vi "stabilizePress_06.vi"() -> ()   [LabVIEW 2011]
uses:
  <vilib>/Analysis/NI_AALPro.lvlib
panel:
  out "dt_array":dbl[](array[numeric])
  out "P_i+1 (torr)":dbl=20.01 caption="P_i+1(torr)" format="%.2f"
  out "Polynomial Coefficients":dbl[](array[numeric])
  in  "n":dbl
  in  "points":i32
  out "P array":dbl[](array[numeric])
  out "t array":dbl[](array[numeric])
  in  "i":u16
  out "tElaps":dbl=32.29700000002049
  in  "dT_fit(s)":dbl=1.0
  in  "tTotal(s)":dbl=30.0
  out "XY Graph":cluster{"Value":dbl[], "Value":dbl[]}(graph)={"Value"=[1.5420000000158325, 3.0790000000270084, 4.619000000006054, 6.157000000006519, 7.695000000006985, 9.23300000000745, 10.772999999986496, 12.309999999997672, 13.847000000008848, 15.386999999987893, 16.92399999999907, 18.462999999988824, 19.99900000001071, 21.53499999997439, 23.07400000002235, 24.61099999997532, 26.147999999986496, 27.68499999999767, 29.222999999998137, 30.760999999998603, 32.29700000002049], "Value"=[16.36, 19.38, 18.91, 17.669999999999998, 16.93, 17.98, 18.610000000000003, 18.83, 19.259999999999998, 19.459999999999997, 19.55, 19.71, 19.91, 19.939999999999998, 19.92, 19.939999999999998, 19.959999999999997, 19.959999999999997, 19.950000000000003, 19.950000000000003, 20.01]}
  out "tune Setpoint(torr)":dbl=20.0
  out "stabilize done":bool=TRUE
  in  "tExp(s)":dbl=15.0
  out "Set Point (torr)":dbl=20.0 format="%.2f"
  out "Setpoint Index":string="C"
  out "Setpoint Index control":u16(ring)=2 caption="Setpoint" items=["A", "B", "C", "D"]
  out "t_0":dbl=343263.848
  in  "time done (s)":dbl
  out "Wait to set":bool
  out "IO error":errorcluster={"status"=FALSE, "code"=1073676418, "source"="VISA Close in WriteAdaptorr04.vi->writeSetPoint_01.vi->stabilizePress_05.vi"}
  in  "stop":bool
  out "Pi (torr)":dbl=20.01 caption="P(torr)" format="%.2f"
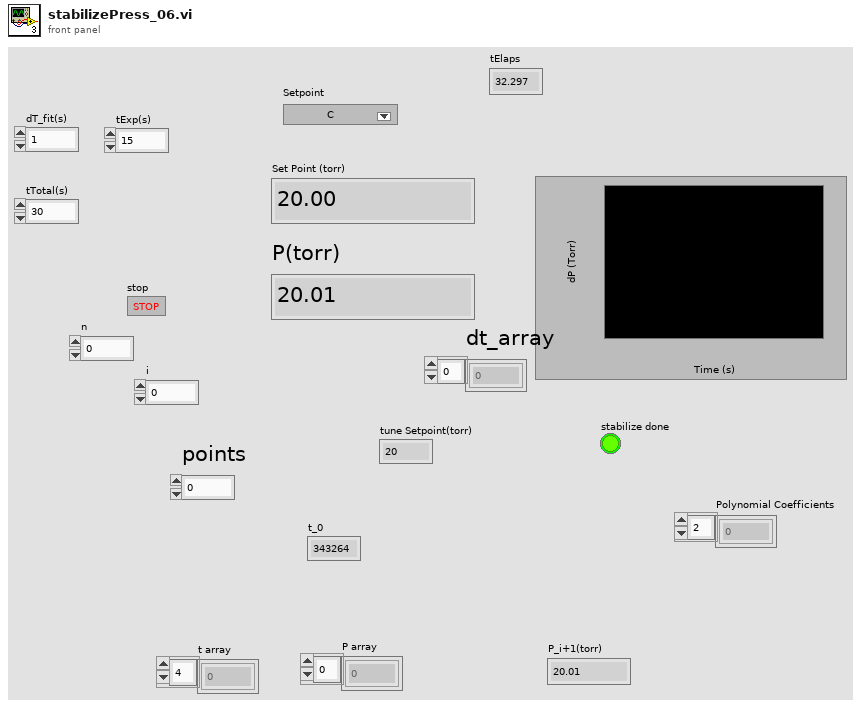
[diagram p1: front panel]
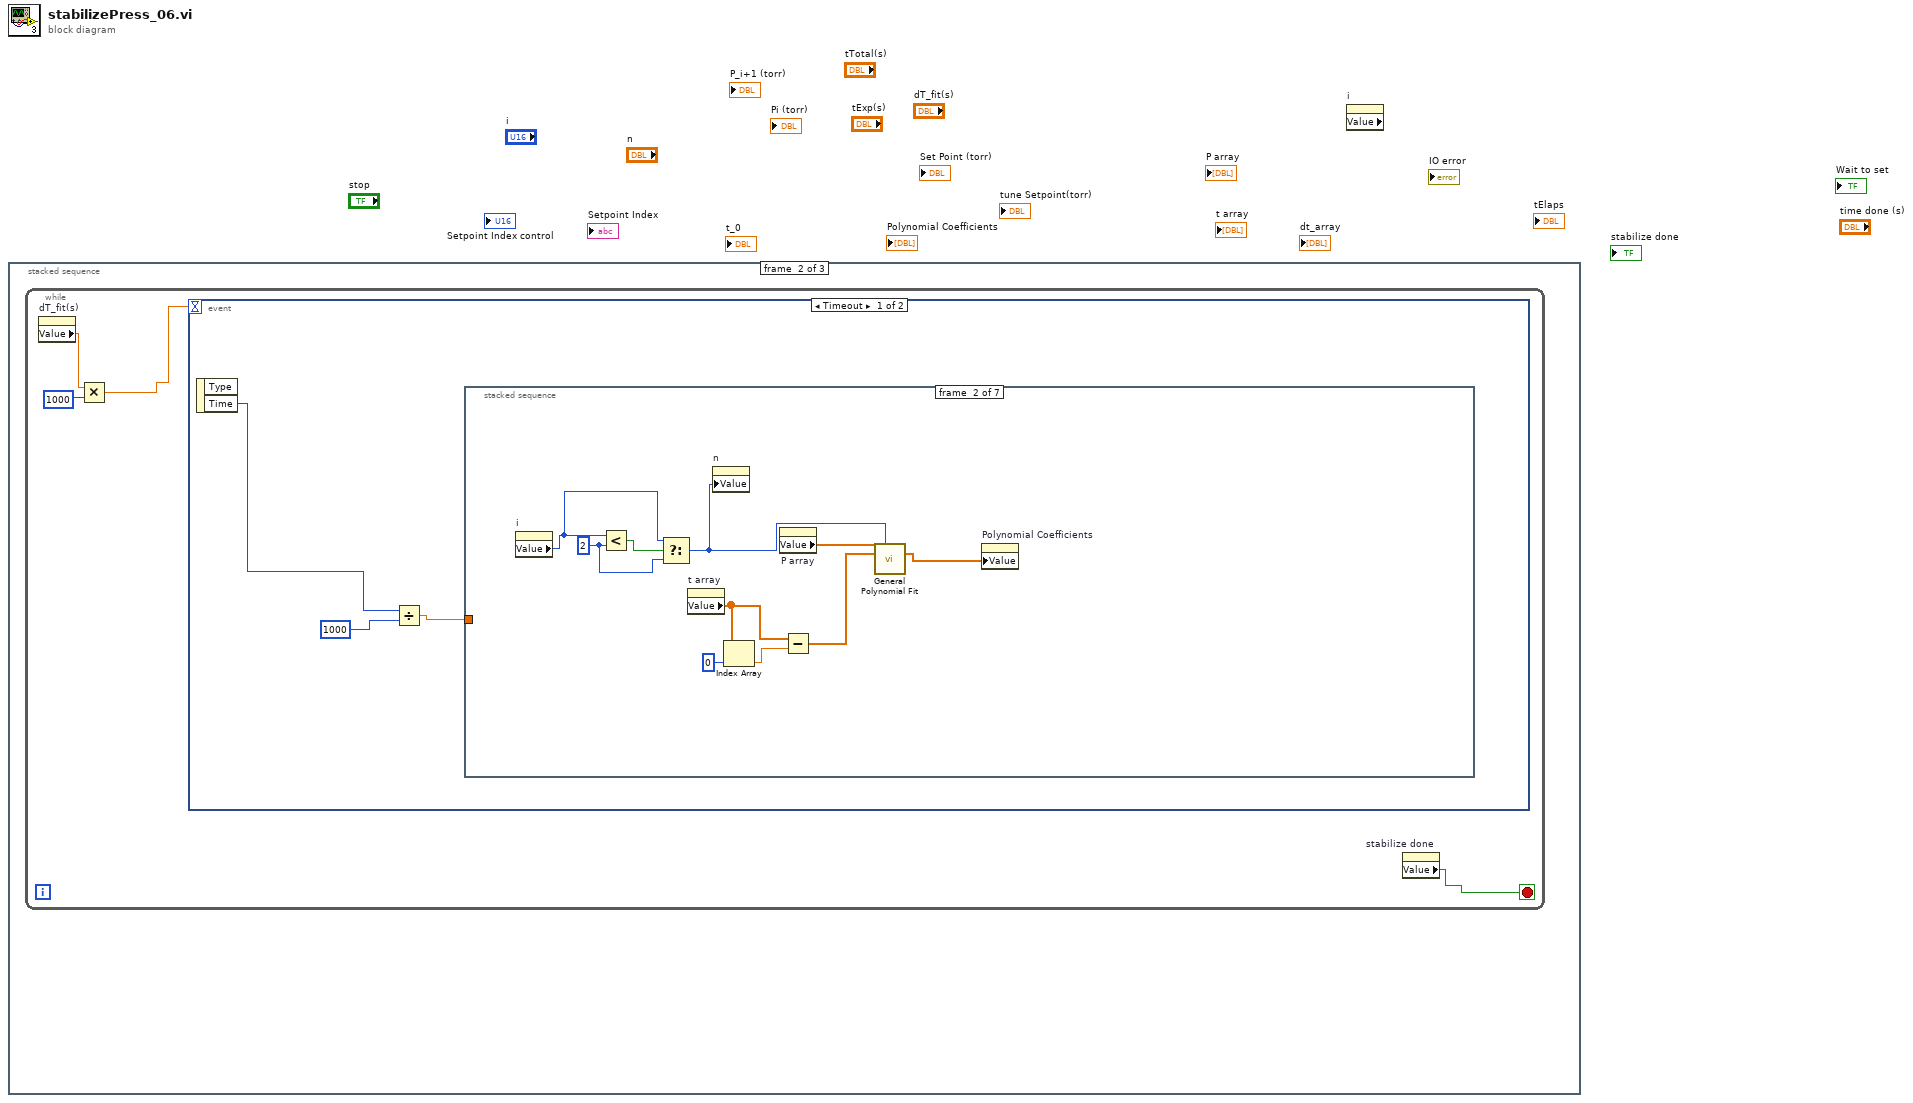
[diagram p0: block diagram]
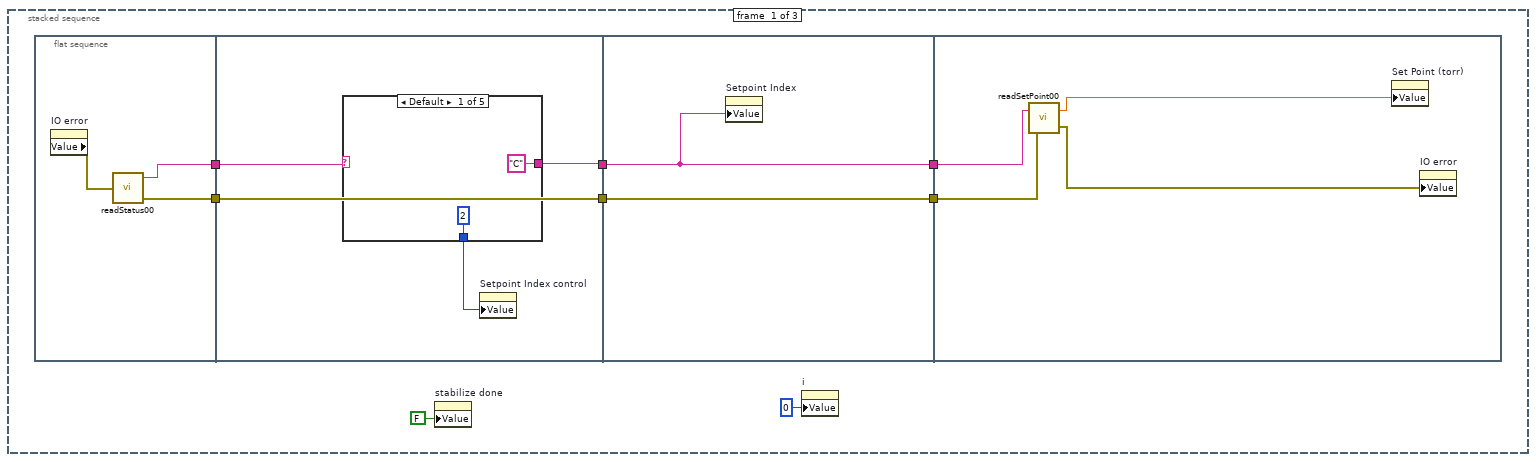
[diagram p2: hidden frame]
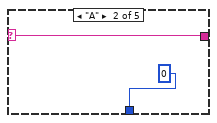
[diagram p3: hidden frame]
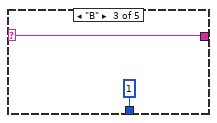
[diagram p4: hidden frame]
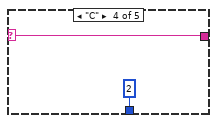
[diagram p5: hidden frame]
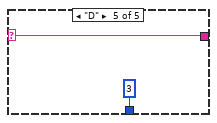
[diagram p6: hidden frame]
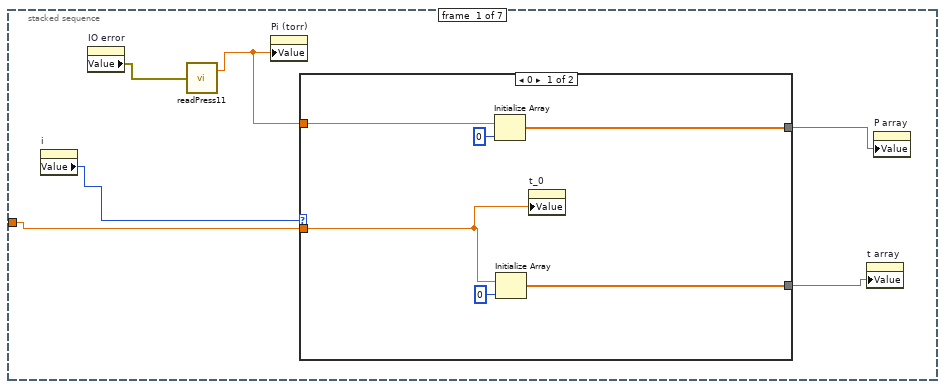
[diagram p7: hidden frame]
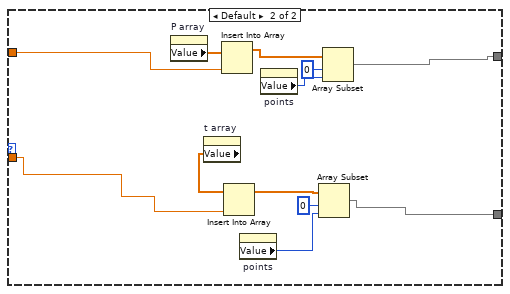
[diagram p8: hidden frame]
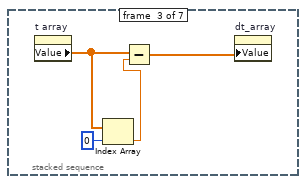
[diagram p9: hidden frame]
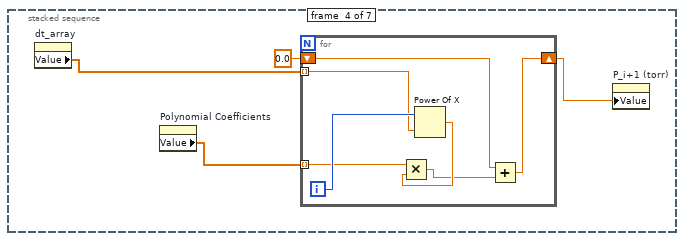
[diagram p10: hidden frame]
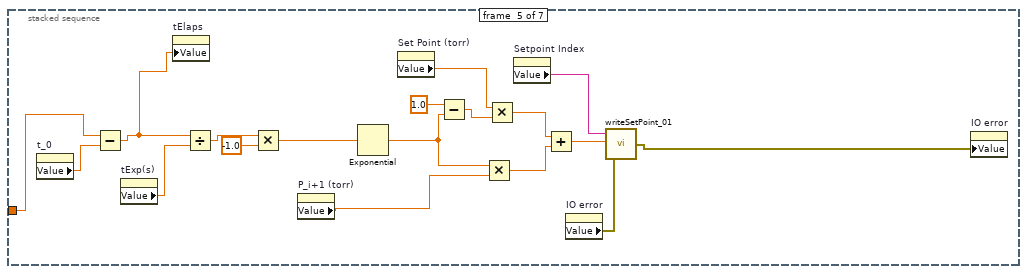
[diagram p11: hidden frame]
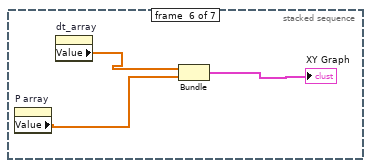
[diagram p12: hidden frame]
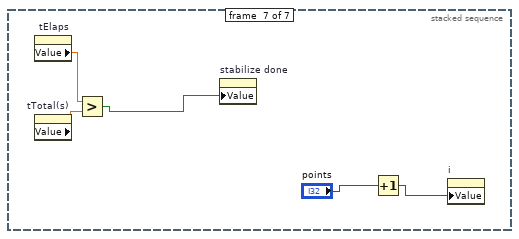
[diagram p13: hidden frame]
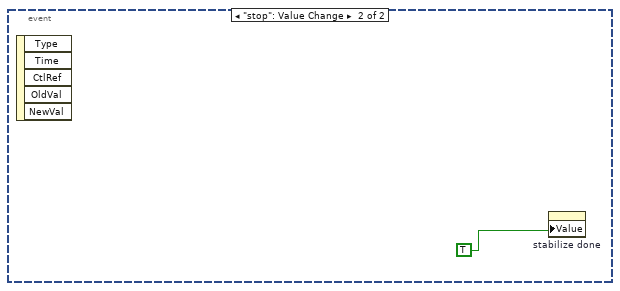
[diagram p14: hidden frame]
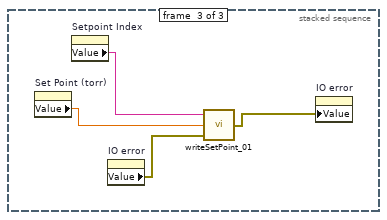
[diagram p15: hidden frame]
diagram:
  n1 = stacked-sequence {
    frame #0 {
      n2 = flat-sequence {
        tunnel: [w10] -> w8
        tunnel: [w9] -> w7
        tunnel: w8 -> [w14]
        tunnel: [w13] -> w6
        tunnel: w7 -> [w15]
        tunnel: [w15] -> w5
        tunnel: w6 -> [w26]
        tunnel: [w26] -> w4
        tunnel: w5 -> [w27]
        tunnel: [w27] -> w3
        tunnel: w4 -> [w31]
        tunnel: w3 -> [w30]
        frame #0 {
          n3 = property on="IO error" class="Clust (strict)"() -> ("Value"=w11:errorcluster)  [unwired: 2 in, 2 out]
          n4 = call "readStatus00.vi"("error in"=w11) -> ("Setpoint"=w10:string, "error out"=w9:errorcluster)  [unwired: 1 out]
        }
        frame #1 {
          n5 = case shown="Default" w14 {
            selector: w14 -> [_ w19 w20 w22 w24]
            tunnel: ["C" w19 w20 w22 w24] -> w13
            tunnel: [u16 2 ("Ring") u16 0 ("Ring") u16 1 ("Ring") u16 2 ("Ring") u16 3 ("Ring")] -> w12
            frame Default {
            }
            frame "A" {
            }
            frame "B" {
            }
            frame "C" {
            }
            frame "D" {
            }
          }
          n6 = property on="Setpoint Index control" class="Ring (strict)"("Value"=w12) -> ()  [unwired: 2 in, 2 out]
        }
        frame #2 {
          n7 = property on="Setpoint Index" class="Str"("Value"=w26) -> ()  [unwired: 2 in, 2 out]
        }
        frame #3 {
          n8 = call "readSetPoint00.vi"("error in"=w30, "Setpoint"=w31) -> ("error out"=w29:errorcluster, "P"=w28:dbl)
          n9 = property on="Set Point (torr)" class="DigNum (strict)"("Value"=w28) -> ()  [unwired: 2 in, 2 out]
          n10 = property on="IO error" class="Clust (strict)"("Value"=w29) -> ()  [unwired: 2 in, 2 out]
        }
      }
      n11 = property on="stabilize done" class="Bool (strict)"("Value"=FALSE ("fit done")) -> ()  [unwired: 2 in, 2 out]
      n12 = property on="i" class="DigNum (strict)"("Value"=u16 0 ("i")) -> ()  [unwired: 2 in, 2 out]
    }
    frame #1 {
      n13 = while {
        stop <- w32 stop-if-true
        n14 = property on="dT_fit(s)" class="DigNum (strict)"() -> ("Value"=w34:dbl)  [unwired: 2 in, 2 out]
        n15 = Multiply(x=w34, y=u32 1000) -> (x*y=w33:dbl)
        n16 = event shown="[0] Timeout" {
          selector: _ -> [_ _]
          dyn-events: _ -> [_ _]
          timeout: w33 -> [_ _]
          event Timeout {
            n17 = event-data() -> ("Time"=w36:u32)  [unwired: 1 in, 1 out]
            n18 = Divide(x=w36, y=i64 1000) -> (x/y=w37:dbl)
            n19 = stacked-sequence {
              tunnel: w37 -> [w39 _ _ _ w88 _ _]
              frame #0 {
                n20 = property on="i" class="DigNum (strict)"() -> ("Value"=w43:u16)  [unwired: 2 in, 2 out]
                n21 = property on="IO error" class="Clust (strict)"() -> ("Value"=w44:errorcluster)  [unwired: 2 in, 2 out]
                n22 = call "readPress11.vi"("error in"=w44) -> ("P"=w42:dbl)  [unwired: 1 out]
                n23 = property on="Pi (torr)" class="DigNum (strict)"("Value"=w42) -> ()  [unwired: 2 in, 2 out]
                n24 = case shown="0" w43 {
                  tunnel: w39 -> [w45 w51]
                  tunnel: w42 -> [w49 w62]
                  tunnel: [w47 w53] -> w41
                  tunnel: [w46 w52] -> w40
                  frame 0 {
                    n25 = Initialize Array(w49, 0 ("dimension size")) -> (w47:dbl[])
                    n26 = Initialize Array(w45, 0 ("dimension size")) -> (w46:dbl[])
                    n27 = property on="t_0" class="DigNum (strict)"("Value"=w45) -> ()  [unwired: 2 in, 2 out]
                  }
                  frame Default {
                    n28 = property on="P array" class="Arr (strict)"() -> ("Value"=w61:dbl[])  [unwired: 2 in, 2 out]
                    n29 = property on="t array" class="Arr (strict)"() -> ("Value"=w60:dbl[])  [unwired: 2 in, 2 out]
                    n30 = Insert Into Array(array=w61, new element=w62) -> (w59:dbl[])  [unwired: 1 in]
                    n31 = Insert Into Array(array=w60, new element=w51) -> (w56:dbl[])  [unwired: 1 in]
                    n32 = property on="points" class="DigNum (strict)"() -> ("Value"=w54:i32)  [unwired: 2 in, 2 out]
                    n33 = property on="points" class="DigNum (strict)"() -> ("Value"=w58:i32)  [unwired: 2 in, 2 out]
                    n34 = Array Subset(array=w56, index=0, length=w54) -> (w52:dbl[])
                    n35 = Array Subset(array=w59, index=0, length=w58) -> (w53:dbl[])
                  }
                }
                n36 = property on="t array" class="Arr (strict)"("Value"=w40) -> ()  [unwired: 2 in, 2 out]
                n37 = property on="P array" class="Arr (strict)"("Value"=w41) -> ()  [unwired: 2 in, 2 out]
              }
              frame #1 {
                w63 = u16 2 ("y")
                n38 = property on="i" class="DigNum (strict)"() -> ("Value"=w64:u16)  [unwired: 2 in, 2 out]
                n39 = Less?(x=w64, y=w63) -> (x < y?=w71:bool)
                n40 = Select(t=w64, s=w71, f=w63) -> (s? t:f=w69:u16)
                n41 = property on="t array" class="Arr (strict)"() -> ("Value"=w66:dbl[])  [unwired: 2 in, 2 out]
                n42 = property on="n" class="DigNum (strict)"("Value"=w69) -> ()  [unwired: 2 in, 2 out]
                n43 = Index Array(array=w66, index=0) -> (element=w67:dbl)
                n44 = property on="P array" class="Arr (strict)"() -> ("Value"=w72:dbl[])  [unwired: 2 in, 2 out]
                n45 = Subtract(x=w66, y=w67) -> (x-y=w65:dbl[])
                n46 = call <vilib>:"General Polynomial Fit.vi"("Y"=w72, "polynomial order"=w69, "X"=w65) -> ("Polynomial Coefficients"=w70:dbl[])  [unwired: 9 in, 3 out]
                n47 = property on="Polynomial Coefficients" class="Arr (strict)"("Value"=w70) -> ()  [unwired: 2 in, 2 out]
              }
              frame #2 {
                n48 = property on="t array" class="Arr (strict)"() -> ("Value"=w76:dbl[])  [unwired: 2 in, 2 out]
                n49 = Index Array(array=w76, index=0) -> (element=w74:dbl)
                n50 = Subtract(x=w76, y=w74) -> (x-y=w73:dbl[])
                n51 = property on="dt_array" class="Arr (strict)"("Value"=w73) -> ()  [unwired: 2 in, 2 out]
              }
              frame #3 {
                n52 = property on="dt_array" class="Arr (strict)"() -> ("Value"=w77:dbl[])  [unwired: 2 in, 2 out]
                n53 = property on="Polynomial Coefficients" class="Arr (strict)"() -> ("Value"=w80:dbl[])  [unwired: 2 in, 2 out]
                n54 = for {
                  tunnel: w77 -> [w86] mode=indexing
                  tunnel: w80 -> [w85] mode=indexing
                  shift-right: [w81] -> w78
                  shift-left: 0.0 -> [w82]
                  i -> [w87]
                  n55 = Power Of X(1:w86, 2:w87) -> (0:w84:dbl)
                  n56 = Multiply(x=w85, y=w84) -> (x*y=w83:dbl)
                  n57 = Add(x=w82, y=w83) -> (x+y=w81:dbl)
                }
                n58 = property on="P_i+1 (torr)" class="DigNum (strict)"("Value"=w78) -> ()  [unwired: 2 in, 2 out]
              }
              frame #4 {
                n59 = property on="t_0" class="DigNum (strict)"() -> ("Value"=w105:dbl)  [unwired: 2 in, 2 out]
                n60 = Subtract(x=w88, y=w105) -> (x-y=w90:dbl)
                n61 = property on="tExp(s)" class="DigNum (strict)"() -> ("Value"=w104:dbl)  [unwired: 2 in, 2 out]
                n62 = property on="tElaps" class="DigNum (strict)"("Value"=w90) -> ()  [unwired: 2 in, 2 out]
                n63 = Divide(x=w90, y=w104) -> (x/y=w103:dbl)
                n64 = Multiply(x=w103, y=-1.0) -> (x*y=w101:dbl)
                n65 = property on="P_i+1 (torr)" class="DigNum (strict)"() -> ("Value"=w89:dbl)  [unwired: 2 in, 2 out]
                n66 = Exponential(1:w101) -> (0:w97:dbl)
                n67 = property on="Set Point (torr)" class="DigNum (strict)"() -> ("Value"=w98:dbl)  [unwired: 2 in, 2 out]
                n68 = Subtract(x=1.0, y=w97) -> (x-y=w99:dbl)
                n69 = Multiply(x=w97, y=w89) -> (x*y=w95:dbl)
                n70 = Multiply(x=w98, y=w99) -> (x*y=w96:dbl)
                n71 = property on="Setpoint Index" class="Str"() -> ("Value"=w93:string)  [unwired: 2 in, 2 out]
                n72 = Add(x=w96, y=w95) -> (x+y=w94:dbl)
                n73 = property on="IO error" class="Clust (strict)"() -> ("Value"=w92:errorcluster)  [unwired: 2 in, 2 out]
                n74 = call "writeSetPoint_01.vi"("error in"=w92, "P (Torr)"=w94, "Setpoint"=w93) -> ("error out"=w91:errorcluster)
                n75 = property on="IO error" class="Clust (strict)"("Value"=w91) -> ()  [unwired: 2 in, 2 out]
              }
              frame #5 {
                n76 = property on="P array" class="Arr (strict)"() -> ("Value"=w107:dbl[])  [unwired: 2 in, 2 out]
                n77 = property on="dt_array" class="Arr (strict)"() -> ("Value"=w106:dbl[])  [unwired: 2 in, 2 out]
                n78 = Bundle "Bundle"("Value"=w106, "Value"=w107) -> (→"XY Graph":cluster{"Value":dbl[], "Value":dbl[]})  [unwired: 1 in]
              }
              frame #6 {
                n79 = property on="tElaps" class="DigNum (strict)"() -> ("Value"=w112:dbl)  [unwired: 2 in, 2 out]
                n80 = property on="tTotal(s)" class="DigNum (strict)"() -> ("Value"=w113:dbl)  [unwired: 2 in, 2 out]
                n81 = Greater?(x=w112, y=w113) -> (0:w111:bool)
                n82 = property on="stabilize done" class="Bool (strict)"("Value"=w111) -> ()  [unwired: 2 in, 2 out]
                n83 = Increment(x="points") -> (x+1=w109:i32)
                n84 = property on="i" class="DigNum (strict)"("Value"=w109) -> ()  [unwired: 2 in, 2 out]
              }
            }
          }
          event "stop": Value Change {
            n85 = event-data() -> ()  [unwired: 1 in, 5 out]
            n86 = property on="stabilize done" class="Bool (strict)"("Value"=TRUE ("stabilize done")) -> ()  [unwired: 2 in, 2 out]
          }
        }
        n87 = property on="stabilize done" class="Bool (strict)"() -> ("Value"=w32:bool)  [unwired: 2 in, 2 out]
      }
    }
    frame #2 {
      n88 = property on="Set Point (torr)" class="DigNum (strict)"() -> ("Value"=w118:dbl)  [unwired: 2 in, 2 out]
      n89 = property on="Setpoint Index" class="Str"() -> ("Value"=w117:string)  [unwired: 2 in, 2 out]
      n90 = property on="IO error" class="Clust (strict)"() -> ("Value"=w116:errorcluster)  [unwired: 2 in, 2 out]
      n91 = call "writeSetPoint_01.vi"("error in"=w116, "P (Torr)"=w118, "Setpoint"=w117) -> ("error out"=w115:errorcluster)
      n92 = property on="IO error" class="Clust (strict)"("Value"=w115) -> ()  [unwired: 2 in, 2 out]
    }
  }
  n93 = property on="i" class="DigNum (strict)" props=["Value"]() -> ()  [unwired: 2 in, 3 out]
